vi "train_GAN_G.vi"(0 "error in (no error)":errorcluster, 1 "ptr":i64, 3 "gamma":sgl, 4 "eta":sgl, 5 "lambda":sgl, 6 "input":sgl[][](array[numeric]), 7 "deltaMatrix":sgl[][](array[numeric]), 8 "RMSProp":bool, 9 "batch_update":u32, 10 "weight_normalization":bool, 11 "first_layer":u32, 12 "adam":bool, 13 "last_layer":u32) -> (14 "error out":errorcluster, 15 "ptr out":i64, 18 "generated":sgl[][](array[numeric]))   [LabVIEW 2016]
uses:
  Users/jg754/Documents/Visual Studio 2015/Projects/CLearn/x64/Release/CLearn.dll
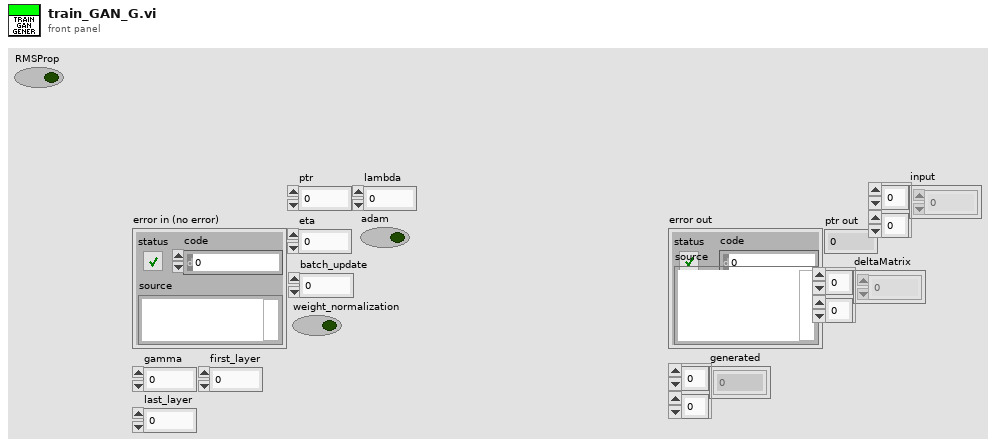
[diagram p1: front panel]
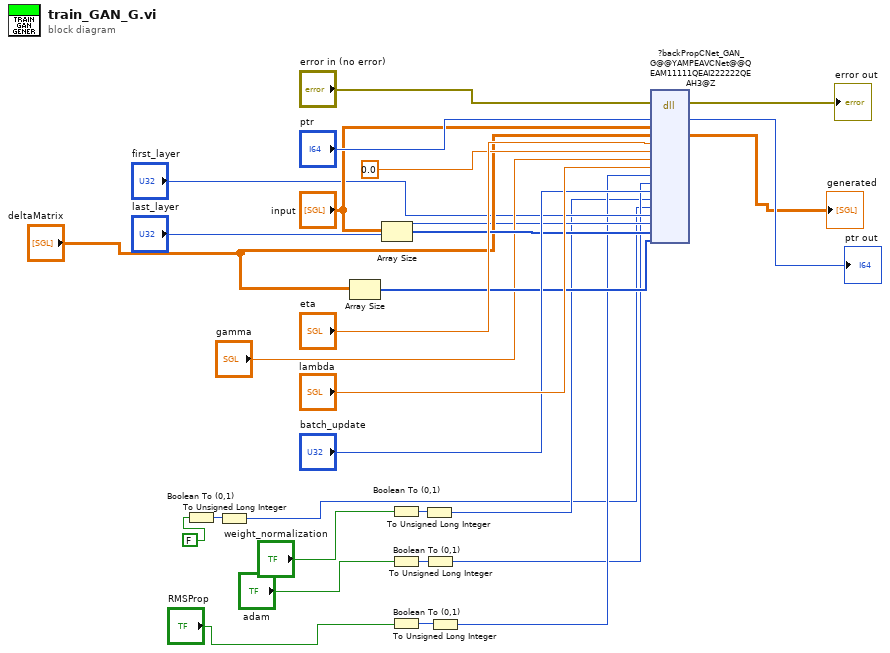
[diagram p0: block diagram]
diagram:
  n1 = Boolean To (0,1)(Boolean=FALSE) -> (0, 1=w4:i16)
  n2 = To Unsigned Long Integer(number=w4) -> (unsigned 32bit integer=w3:u32)
  n3 = Array Size(array="deltaMatrix") -> (size(s)=w14:i32[])
  n4 = Array Size(array="input") -> (size(s)=w16:i32[])
  n5 = Boolean To (0,1)(Boolean="weight_normalization") -> (0, 1=w6:i16)
  n6 = Boolean To (0,1)(Boolean="adam") -> (0, 1=w8:i16)
  n7 = Boolean To (0,1)(Boolean="RMSProp") -> (0, 1=w10:i16)
  n8 = To Unsigned Long Integer(number=w6) -> (unsigned 32bit integer=w5:u32)
  n9 = To Unsigned Long Integer(number=w8) -> (unsigned 32bit integer=w7:u32)
  n10 = To Unsigned Long Integer(number=w10) -> (unsigned 32bit integer=w9:u32)
  n11 = dll-call lib="C:/Users/jg754/Documents/Visual Studio 2015/Projects/CLearn/x64/Release/CLearn.dll" fn="?backPropCNet_GAN_G@@YAMPEAVCNet@@QEAM11111QEAI222222QEAH3@Z"(error in="error in (no error)", "ptr"="ptr", "input"="input", "deltaMatrix"="deltaMatrix", "eta"="eta", "metaEta"=sgl 0.0, "gamma"="gamma", "lambda"="lambda", "RMSprop"=w9, "adam"=w7, "batch_update"="batch_update", "weight_normalization"=w5, "spectral_normalization"=w3, "first_layer"="first_layer", "last_layer"="last_layer", "inFormat"=w16, "deltaFormat"=w14) -> (error out=→"error out":errorcluster, "ptr"=→"ptr out":i64, "deltaMatrix"=→"generated":sgl[][])  [unwired: 17 in, 1 out]
